vi "rs232.vi"() -> ()   [LabVIEW 2015]
uses:
  <vilib>/Instr/_visa.llb/VISA Configure Serial Port (Instr).vi
panel:
  out "error out":errorcluster
  in  "string to write":string="*IDN?"
  in  "stop":bool
  in  "read":bool=TRUE
  in  "write":bool=TRUE
  out "read string":string
  out "actual bytes read":u32
  in  "XON Character":u8=17 format="%.0x"
  in  "XOFF Character":u8=19 format="%.0x"
  in  "flow control":u16(ring) items=["None"=0, "XON/XOFF"=1, "RTS/CTS"=2, "DTR/DSR"=4]
  in  "End write with termination character?":bool=TRUE
  in  "termination char\n(0xA = '\\n' = LF)":u8=10 format="%.0x"
  in  "End read on termination character?":bool=TRUE
  in  "timeout (ms)":u32=10000
  in  "stop bits":u16(ring)=10 items=["1.0"=10, "1.5"=15, "2.0"=20]
  in  "parity":u16(ring) items=["None", "Odd", "Even", "Mark", "Space"]
  in  "data bits":u16=8 min=5 max=8 step=1
  in  "VISA resource name":refnum<visa-resource-name>="COM1"
  in  "baud rate":u32=9600
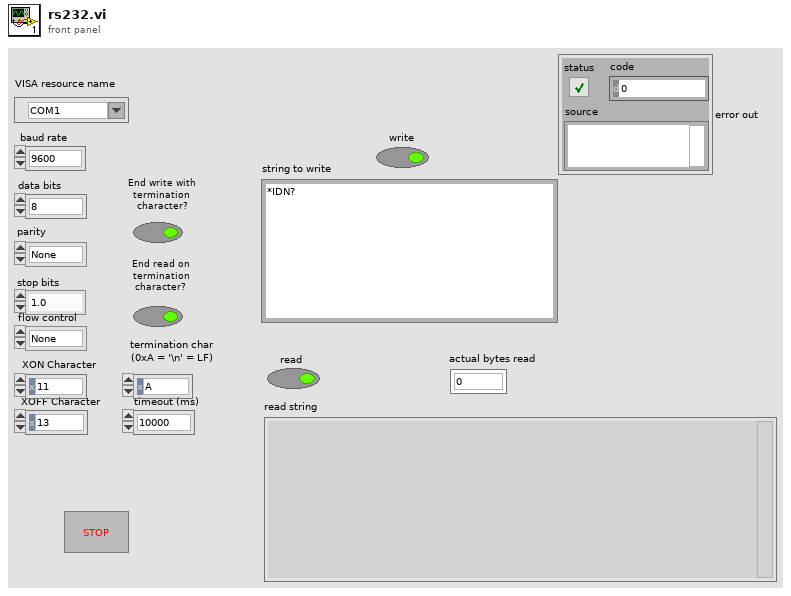
[diagram p1: front panel]
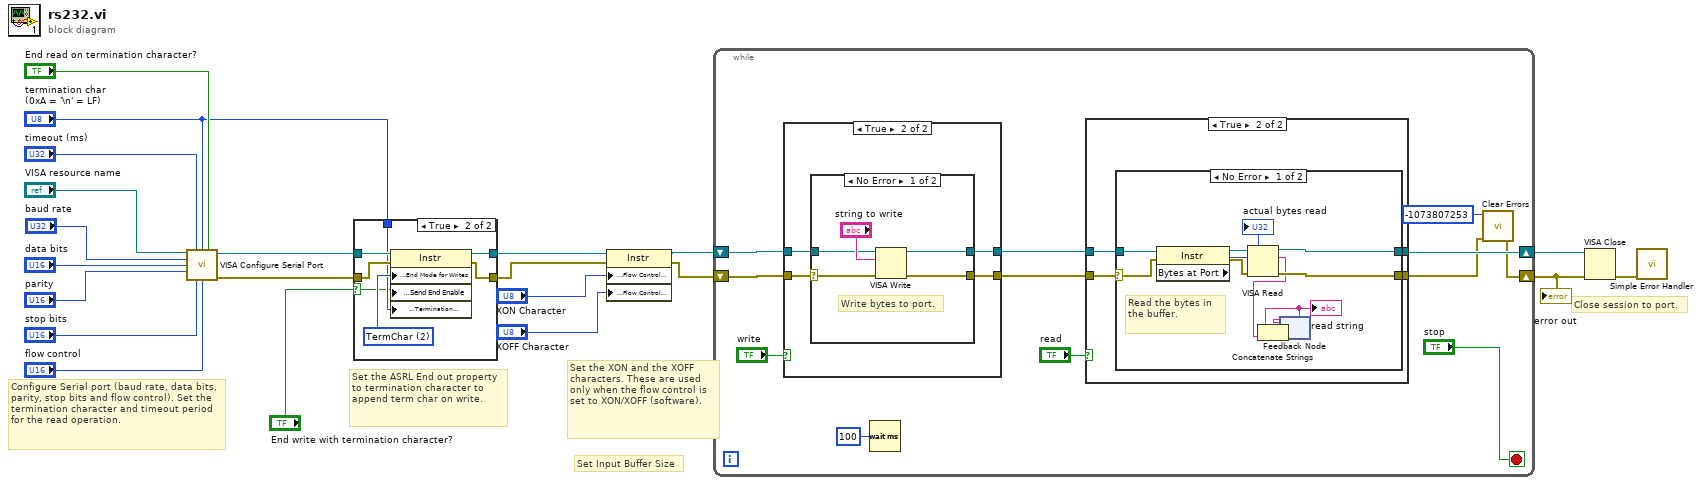
[diagram p0: block diagram]
diagram:
  # "Close session to port."
  # "Set the XON and the XOFF characters. These are used only when the flow control is set to XON/XOFF (software)."
  # "Configure Serial port (baud rate, data bits, parity, stop bits and flow control). Set the termination character and timeout period for the read operation."
  # "Set Input Buffer Size"
  # "Set the ASRL End out property to termination character to append term char on write."
  n1 = call-poly "VISA Configure Serial Port"("VISA resource name"="VISA resource name", "timeout (10sec)"="timeout (ms)", "termination char\n(0xA = '\\n' = LF)"="termination char\n(0xA = '\\n' = LF)", "Enable Termination\nChar (T)"="End read on termination character?", "baud rate (9600)"="baud rate", "data bits (8)"="data bits", "parity (0:none)"="parity", "stop bits (10: 1 bit)"="stop bits", "flow control (0:none)"="flow control") -> ("VISA resource name out"=w8:refnum<visa-resource-name>, "error out"=w9:errorcluster)  [unwired: 1 in, 4 out]
  n2 = case shown="True" "End write with termination character?" {
    selector: "End write with termination character?" -> [_ w24]
    tunnel: w8 -> [w22 w30]
    tunnel: w9 -> [w23 w29]
    tunnel: [w22 w28] -> w7
    tunnel: [w23 w27] -> w6
    tunnel: "termination char\n(0xA = '\\n' = LF)" -> [_ w25]
    frame False {
    }
    frame True {
      w26 = u16 2 items=["None", "LastBit", "TermChar", "Break"] ("Serial Settings:Serial End Mode for Writes")
      n3 = property class="Instr"(reference=w30, error in=w29, "Serial Settings:End Mode for Writes"=w26, "Message Based Settings:Send End Enable"=w24, "Message Based Settings:Termination Character"=w25) -> (reference out=w28:refnum<visa-resource-name>, error out=w27:errorcluster)
    }
  }
  n4 = property class="Instr"(reference=w7, error in=w6, "Serial Settings:Flow Control XON Character"="XON Character", "Serial Settings:Flow Control XOFF Character"="XOFF Character") -> (reference out=w2:refnum<visa-resource-name>, error out=w1:errorcluster)
  n5 = while {
    shift-right: [w38] -> w4
    shift-left: w2 -> [w37]
    shift-right: [w32] -> w3
    shift-left: w1 -> [w36]
    stop <- "stop" stop-if-true
    n6 = case shown="True" "write" {
      tunnel: [w44 w48] -> w41
      tunnel: [w43 w47] -> w40
      tunnel: w37 -> [w44 w46]
      tunnel: w36 -> [w43 w45]
      frame False {
      }
      frame True {
        n7 = case shown="No Error" w45 {
          selector: w45 -> [w49 w55]
          tunnel: [w53 w54] -> w48
          tunnel: [w52 w55] -> w47
          tunnel: w46 -> [w50 w54]
          frame No Error {
            # "Write bytes to port."
            n8 = VISA Write(VISA resource name=w50, write buffer="string to write", error in (no error)=w49) -> (VISA resource name out=w53:refnum<visa-resource-name>, error out=w52:errorcluster)  [unwired: 1 out]
          }
          frame Error {
          }
        }
      }
    }
    n9 = Wait (ms)(milliseconds to wait=u32 100) -> ()  [unwired: 1 out]
    n10 = case shown="True" "read" {
      tunnel: w40 -> [w56 w59]
      tunnel: w41 -> [w57 w58]
      tunnel: [w56 w61] -> w33
      tunnel: [w57 w60] -> w38
      frame False {
      }
      frame True {
        n11 = case "Read bytes from port." shown="No Error" w59 {
          selector: w59 -> [w67 w73]
          tunnel: [w71 w73] -> w61
          tunnel: [w72 w74] -> w60
          tunnel: w58 -> [w68 w74]
          frame No Error {
            # "Read the bytes in the buffer."
            n12 = property class="Instr"(reference=w68, error in=w67) -> (reference out=w66:refnum<visa-resource-name>, error out=w65:errorcluster, "Bytes at Port"=w69:u32)
            n13 = VISA Read(VISA resource name=w66, byte count=w69, error in (no error)=w65) -> (VISA resource name out=w72:refnum<visa-resource-name>, read buffer=w64:string, return count=→"actual bytes read":u32, error out=w71:errorcluster)
            n14 = feedback #1() -> (w62:string)  [unwired: 1 in]
            "read string" <- w62
            n15 = Concatenate Strings(w62, w64) -> (w63:string)
            n16 = feedback-in #1(w63) -> ()
          }
          frame Error {
            # "Error occurred \nreading Bytes at \nSerial Port"
          }
        }
      }
    }
    n17 = call <vilib>:"Clear Errors.vi"("error in (no error)"=w33, "specific error code to clear (0: all)"=-1073807253) -> ("error out"=w32:errorcluster)  [unwired: 4 in, 1 out]
  }
  "error out" <- w3
  n18 = VISA Close(VISA resource name=w4, error in (no error)=w3) -> (error out=w5:errorcluster)
  n19 = call <vilib>:"Simple Error Handler.vi"("error in (no error)"=w5) -> ()  [unwired: 1 in, 8 out]
